vi "Configure Output State.vi"(7 "Enable Output (T: Enable)":bool=TRUE, 8 "error in (no error)":errorcluster, 11 "VISA resource name":refnum<visa-resource-name>) -> (0 "error out":errorcluster, 3 "VISA resource name out":refnum<visa-resource-name>)   [LabVIEW 2021, in "BK Precision 169XB.lvlib"]
doc: "Configures output voltage level, channel, and enables or disables the output of the power supply."
uses:
  BK Precision 169XB.lvlib
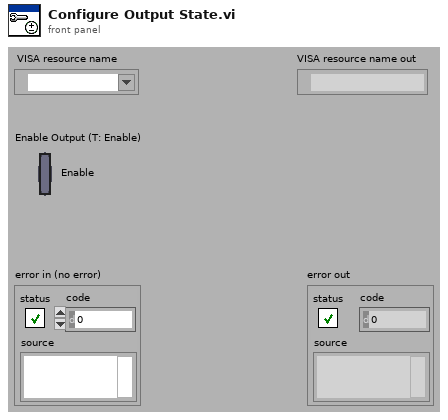
[diagram p1: front panel]
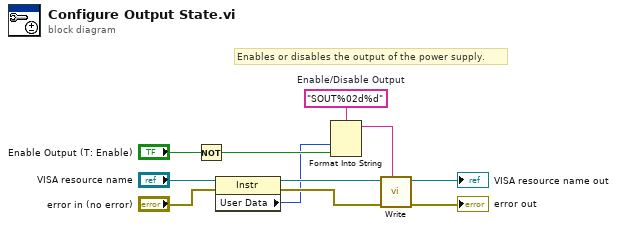
[diagram p0: block diagram]
diagram:
  w11 = "SOUT%02d%d"  # Enable/Disable Output
  # "Enables or disables the output of the power supply."
  n1 = Not(x="Enable Output (T: Enable)") -> (.not. x?=w7:bool)
  n2 = property class="Instr"(reference="VISA resource name", error in="error in (no error)") -> (reference out=w3:refnum<visa-resource-name>, error out=w4:errorcluster, "User Data"=w1:u32)
  n3 = Format Into String(format string=w11, w1, w7) -> (resulting string=w6:string)  [unwired: 2 in, 1 out]
  n4 = call "Write.vi"("Input String"=w6, "error in (no error)"=w4, "VISA resource name"=w3) -> ("error out"=→"error out":errorcluster, "VISA resource name out"=→"VISA resource name out":refnum<visa-resource-name>)  [unwired: 6 in, 1 out]
